vi "Get Target Data.vi"() -> (4 "Yellow":dbl[](array[numeric]), 6 "Green":dbl[](array[numeric]), 8 "Red":dbl[](array[numeric]), 10 "x angle":u16, 15 "y angle":u16)   [LabVIEW 2012]
panel:
  in  "Color 3":string(combo)="RED"
  in  "Color 2":string(combo)="GREEN"
  out "Val":bool
  in  "Color":string(combo)="YELLOW"
  in  "variables":string[](array[string])=["HORIZ_ANGLE", "VERT_ANGLE", "DISTANCE"]
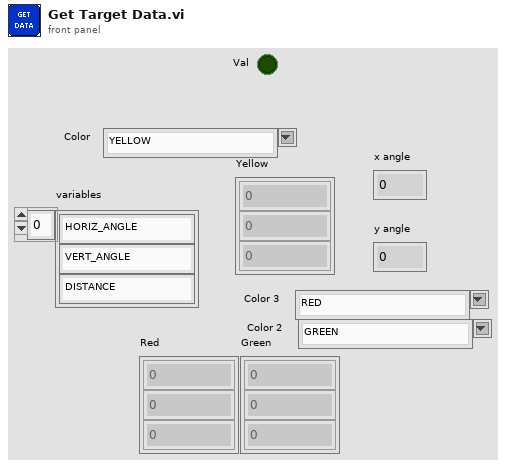
[diagram p1: front panel]
types:
  T1 = typedef "WPI_ServoDeviceRef.ctl" = cluster{"DeviceStatus":errorcluster, "Digital Module":T2, "PWM Channel":T3, "DeadBand":T4}
  T2 = typedef "FPGA_TypedefDigitalModule.ctl" = enum16{"Digital Module 1", "Digital Module 2"}
  T3 = typedef "FPGA_DIOPWMChannel.ctl" = enum8{"PWM 1", "PWM 2", "PWM 3", "PWM 4", "PWM 5", "PWM 6", "PWM 7", "PWM 8", "PWM 9", "PWM 10", "Invalid"}
  T4 = typedef "WPI_PWMDeadband.ctl" = cluster{"Name":string, "maxPositivePwm":i32, "minPositivePwm":i32, "centerPwm":i32, "maxNegativePwm":i32, "minNegativePwm":i32, "angularRange":u16}
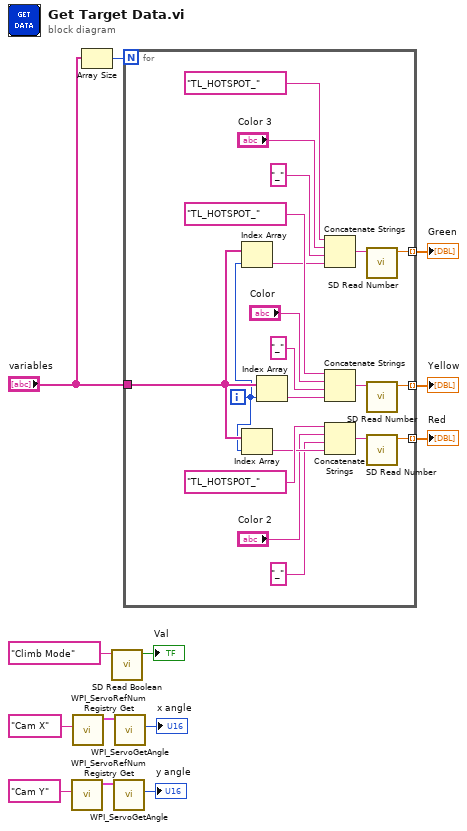
[diagram p0: block diagram]
diagram:
  n1 = call <vilib>:"WPI_ServoRefNum Registry Get.vi"("refnum name"="Cam Y") -> ("ServoDeviceRef"=w5:T1)  [unwired: 9 in, 1 out]
  n2 = call <vilib>:"WPI_ServoRefNum Registry Get.vi"("refnum name"="Cam X") -> ("ServoDeviceRef"=w8:T1)  [unwired: 9 in, 1 out]
  n3 = Array Size(array="variables") -> (size(s)=w13:i32)
  n4 = call <vilib>:"SD Read Boolean.vi"("Name"="Climb Mode") -> ("Boolean"=→"Val":bool)  [unwired: 8 in, 2 out]
  n5 = call <vilib>:"WPI_ServoGetAngle.vi"("ServoDeviceRef"=w5) -> ("Angle"=→"y angle":u16)  [unwired: 7 in, 2 out]
  n6 = call <vilib>:"WPI_ServoGetAngle.vi"("ServoDeviceRef"=w8) -> ("Angle"=→"x angle":u16)  [unwired: 7 in, 2 out]
  n7 = for {
    N: w13 -> [_]
    tunnel: "variables" -> [w17]
    tunnel: [w31] -> w11 mode=indexing
    tunnel: [w22] -> w2 mode=indexing
    tunnel: [w15] -> w1 mode=indexing
    i -> [w14]
    n8 = Index Array(array=w17, index=w14) -> (element=w20:string)
    n9 = Index Array(array=w17, index=w14) -> (element=w26:string)
    n10 = Index Array(array=w17, index=w14) -> (element=w30:string)
    n11 = Concatenate Strings("TL_HOTSPOT_" ("Name"), "Color 3", "_" ("string"), w20) -> (w16:string)
    n12 = Concatenate Strings("TL_HOTSPOT_" ("Name"), "Color", "_" ("string"), w30) -> (w32:string)
    n13 = Concatenate Strings("TL_HOTSPOT_" ("Name"), "Color 2", "_" ("string"), w26) -> (w23:string)
    n14 = call <vilib>:"SD Read Number.vi"("Name"=w16) -> ("Numeric"=w15:dbl)  [unwired: 8 in, 2 out]
    n15 = call <vilib>:"SD Read Number.vi"("Name"=w32) -> ("Numeric"=w31:dbl)  [unwired: 8 in, 2 out]
    n16 = call <vilib>:"SD Read Number.vi"("Name"=w23) -> ("Numeric"=w22:dbl)  [unwired: 8 in, 2 out]
  }
  "Yellow" <- w11
  "Red" <- w2
  "Green" <- w1
